vi "InitializePanelValues.vi"(11 "Experiment State in":T1={"error"={"status"=FALSE, "code"=0, "source"=""}, "Digitizer DAQmx Tasks"={"TaskArray"=[]}, "Digitizer Settings"={"Channel Settings"=[], "Card Settings"=[]}, "Synchronization Settings"={"Synchronizer 0"="", "source terminal"="", "Synchronizer 1"="PXI1Slot2"}, "Digitizer Data"=[], "Next Shot#"="", "System Message"="", "User Shot Notes"="", "Timing Settings"={"Timing Card Settings"=[], "Timing Channel Settings"=[]}, "Timing Tasks"={"TaskArray"=[]}, "Tree"="", "Time Card/Channels"=[], "DAQ Card/Channels"=[], "Program Version"="", "RIO Settings"={"Channel Settings"=[], "Card Settings"=[]}, "RIO References"={"Reference Array"=[]}, "RIO Data"={"RIO Deleaved Data"=[], "Raw Readout"=[]}} {"RIO Settings"."Card Settings"."Sample Rate" format="%#_3p"; "Timing Settings"."Timing Channel Settings"."FrontPanelTime" format="%.3p"; "Timing Settings"."Timing Channel Settings"."Pulse width (s)" format="%.3p"; "Timing Settings"."Timing Channel Settings"."Delay (s)" format="%.3p"; "Digitizer Settings"."Card Settings"."Global Edge Type" items=["Rising"=10280, "Falling"=10171]; "Digitizer Settings"."Card Settings"."Sample Rate" format="%#_3p"}) -> (0 "Initialized DAQ Array":T19(array[cluster]) {"Card Settings"."Start Time" format="%#_3p"; "Card Settings"."End Time" format="%#_3p"; "Card Settings"."Rate" format="%#_3p"}, 1 "Initialized Timing Array":T14[](array[typedef]) {"Timing Sequence"."Dt" format="%_3p"; "Timing Sequence"."Time" format="%_3p"}, 3 "Experiment State out":T1={"error"={"status"=FALSE, "code"=0, "source"=""}, "Digitizer DAQmx Tasks"={"TaskArray"=[]}, "Digitizer Settings"={"Channel Settings"=[], "Card Settings"=[]}, "Synchronization Settings"={"Synchronizer 0"="", "source terminal"="", "Synchronizer 1"="PXI1Slot2"}, "Digitizer Data"=[], "Next Shot#"="", "System Message"="", "User Shot Notes"="", "Timing Settings"={"Timing Card Settings"=[], "Timing Channel Settings"=[]}, "Timing Tasks"={"TaskArray"=[]}, "Tree"="", "Time Card/Channels"=[], "DAQ Card/Channels"=[], "Program Version"="", "RIO Settings"={"Channel Settings"=[], "Card Settings"=[]}, "RIO References"={"Reference Array"=[]}, "RIO Data"={"RIO Deleaved Data"=[], "Raw Readout"=[]}} {"RIO Settings"."Card Settings"."Sample Rate" format="%#_3p"; "Timing Settings"."Timing Channel Settings"."FrontPanelTime" format="%.3p"; "Timing Settings"."Timing Channel Settings"."Pulse width (s)" format="%.3p"; "Timing Settings"."Timing Channel Settings"."Delay (s)" format="%.3p"; "Digitizer Settings"."Card Settings"."Global Edge Type" items=["Rising"=10280, "Falling"=10171]; "Digitizer Settings"."Card Settings"."Sample Rate" format="%#_3p"}, 4 "Next Shot #":i32, 6 "System Message":string, 8 "Program Version":string)   [LabVIEW 2014]
doc: "Initialize values of various front panel boxes. Also initialized is the timing and DAQ card sequencers."
uses:
  Controls/ExperimentStateCluster.ctl
  Controls/DigitizerSettingsChannelSettings.ctl
  Controls/DigitizerSettingsCardSettingsArray.ctl
  Controls/DigitizerSettingsCardSettings.ctl
  Controls/TimingSettings.ctl
  Controls/TimingCardSettings.ctl
  Controls/TimingChannelSettings.ctl
  Controls/RIOSettingsExperimentStateCluster.ctl
  Controls/RIOSettingsChannelSettings.ctl
  Controls/RIOSettingsCardSettingsArray.ctl
  Controls/RIOSettingsCardSettings.ctl
  <vilib>/userdefined/High Color/nirio_resource_hc.ctl
  Controls/RIOData.ctl
  Controls/DAQ Card Channel Array.ctl
  Controls/DAQ Channel Settings.ctl
  Controls/DAQ Card Settings.ctl
  Controls/TimingControl.ctl
  Controls/TimingControlChannel.ctl
panel:
  # "Sampling Rate [1/s]"
  # "Start Time [s]"
  # "End Time [s]"
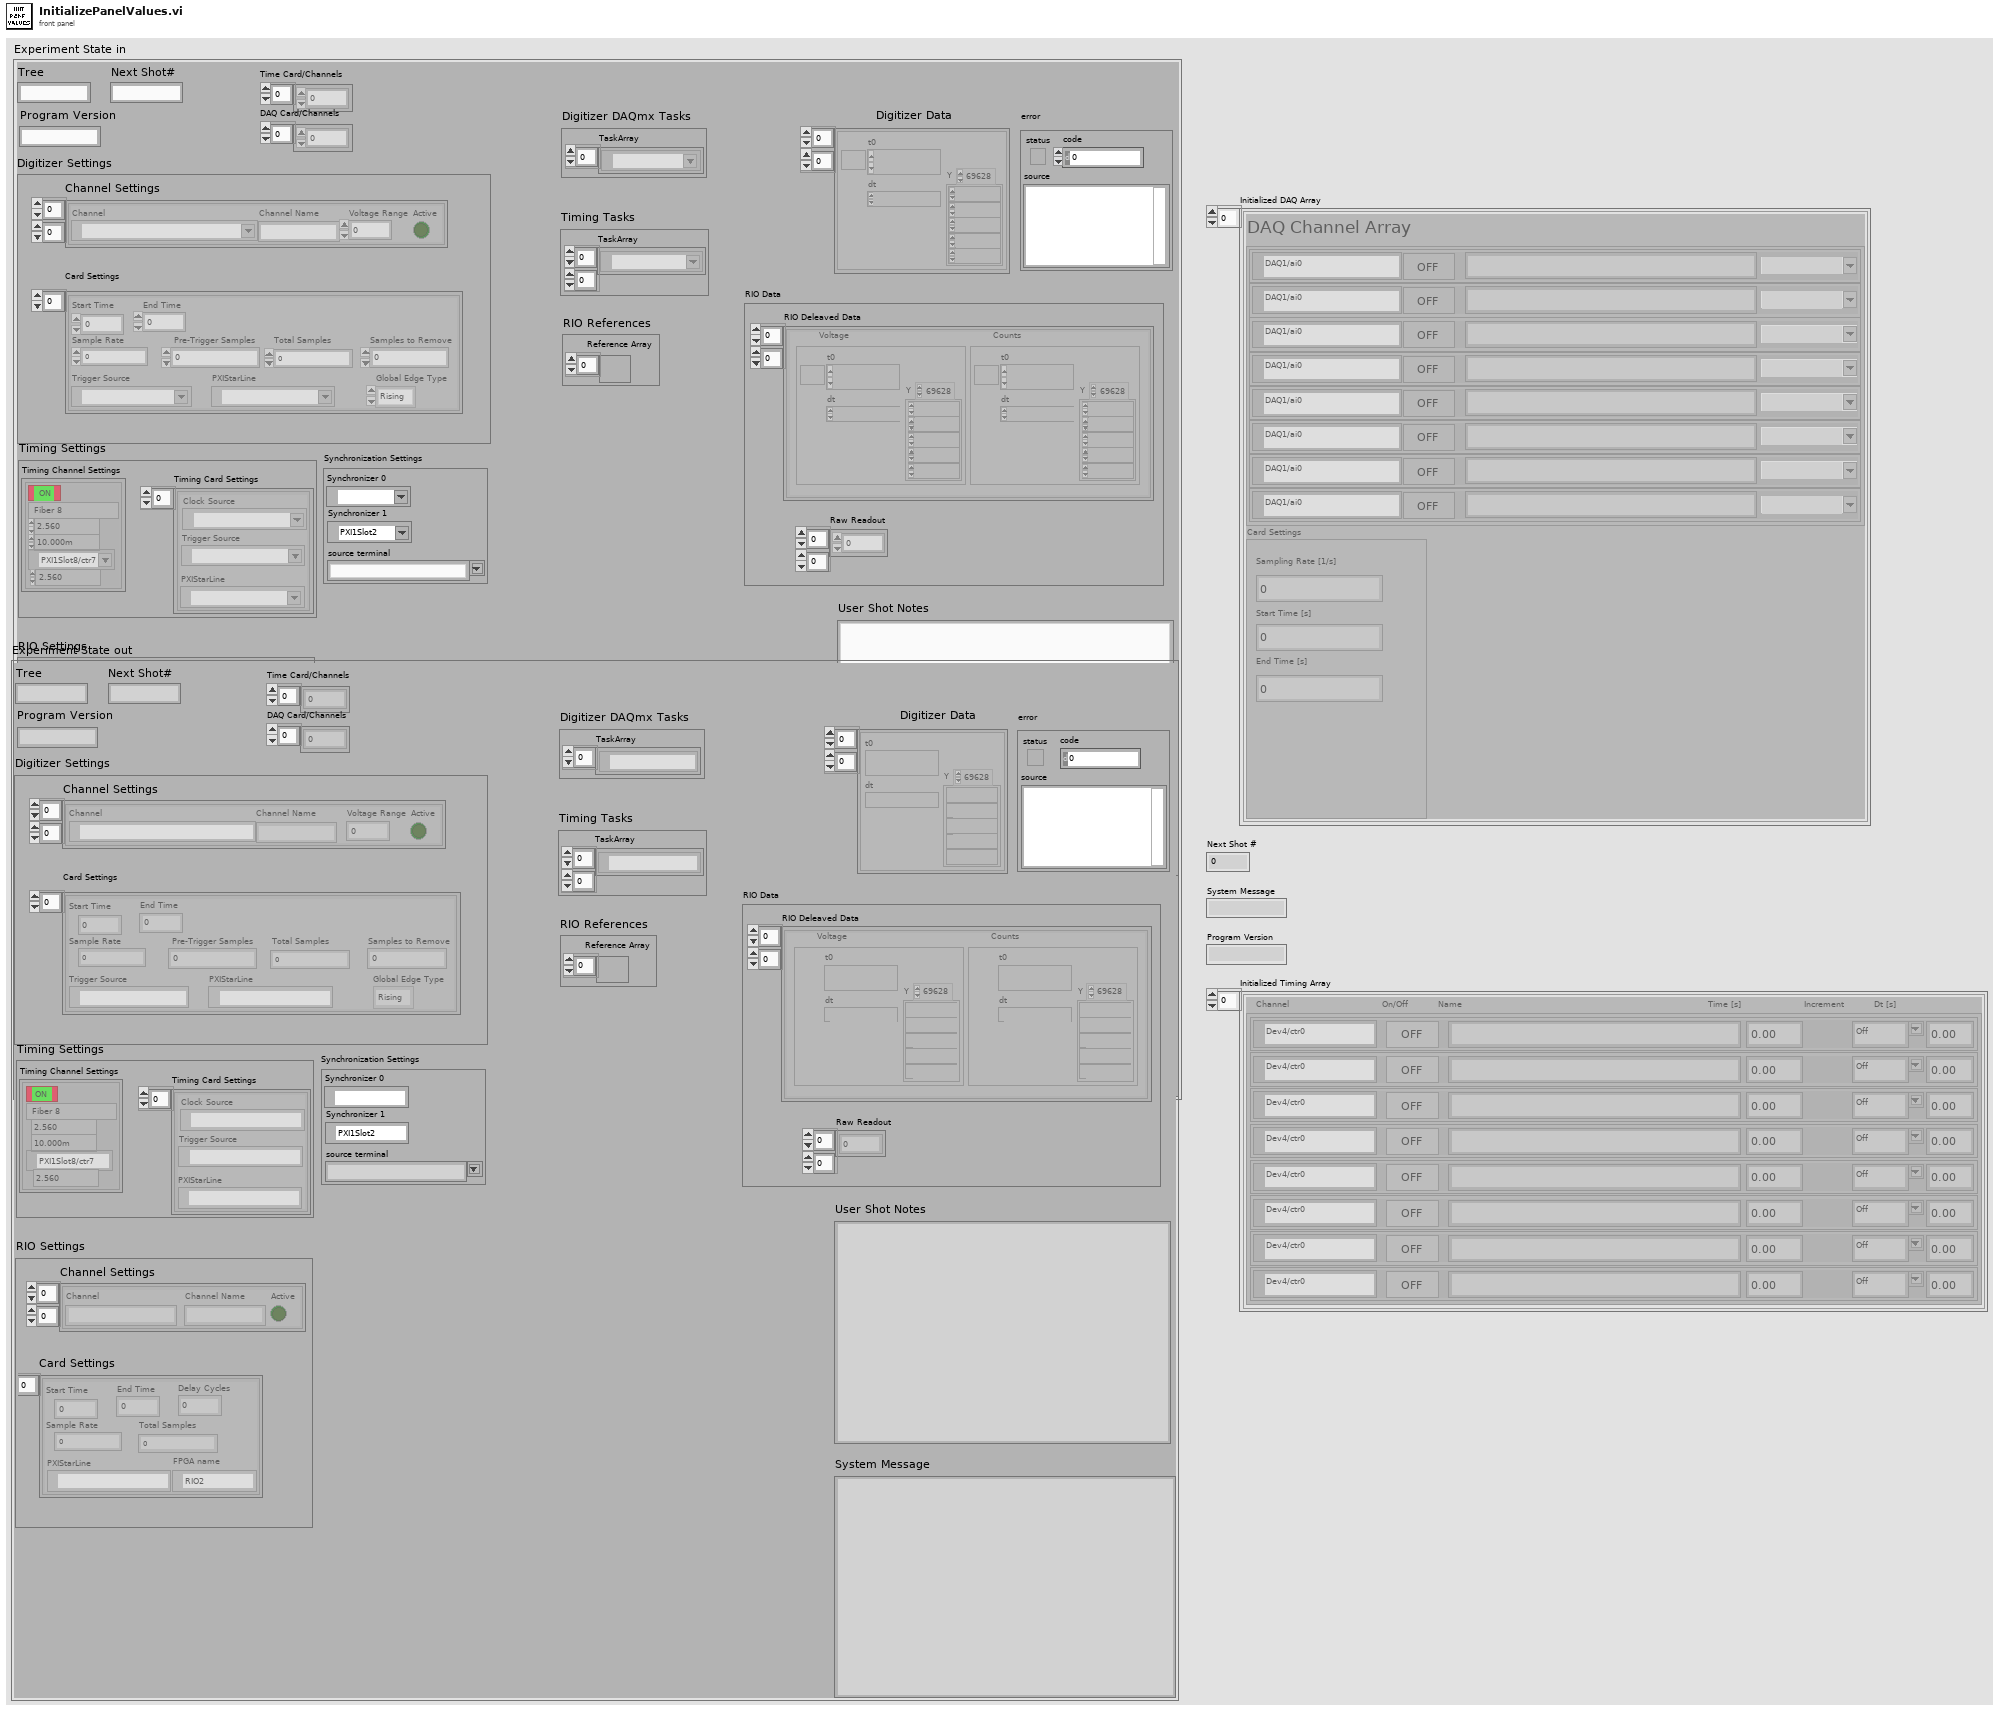
[diagram p1: front panel]
types:
  T1 = typedef "ExperimentStateCluster.ctl" = cluster{"error":errorcluster, "Digitizer DAQmx Tasks":cluster{"TaskArray":refnum<k21>[]}, "Digitizer Settings":cluster{"Channel Settings":T2[][], "Card Settings":T3}, "Synchronization Settings":cluster{"Synchronizer 0":refnum<k15>, "source terminal":string, "Synchronizer 1":refnum<k15>}, "Digitizer Data":waveform(dbl)[][], "Next Shot#":string, "System Message":string, "User Shot Notes":string, "Timing Settings":T5, "Timing Tasks":cluster{"TaskArray":refnum<k21>[][]}, "Tree":string, "Time Card/Channels":i32[], "DAQ Card/Channels":i32[], "Program Version":string, "RIO Settings":T8, "RIO References":cluster{"Reference Array":refnum<k20>[]}, "RIO Data":T13}
  T2 = typedef "DigitizerSettingsChannelSettings.ctl" = cluster{"Channel":tag, "Channel Name":string, "Voltage Range":dbl, "Active":bool}
  T3 = typedef "DigitizerSettingsCardSettingsArray.ctl" = T4[]
  T4 = typedef "DigitizerSettingsCardSettings.ctl" = cluster{"Start Time":dbl, "End Time":dbl, "Sample Rate":dbl, " Pre-Trigger Samples":u32, "Total Samples":i32, "Samples to Remove":u32, "Trigger Source":tag, "Global Edge Type":i32, "PXIStarLine":tag}
  T5 = typedef "TimingSettings.ctl" = cluster{"Timing Card Settings":T6[], "Timing Channel Settings":T7[][]}
  T6 = typedef "TimingCardSettings.ctl" = cluster{"Trigger Source":tag, "Clock Source":tag, "PXIStarLine":tag}
  T7 = typedef "TimingChannelSettings.ctl" = cluster{"Delay (s)":dbl, "Pulse width (s)":dbl, "Active":bool, "Channel Name":string, "counter":tag, "FrontPanelTime":dbl}
  T8 = typedef "RIOSettingsExperimentStateCluster.ctl" = cluster{"Channel Settings":T9[][], "Card Settings":T10}
  T9 = typedef "RIOSettingsChannelSettings.ctl" = cluster{"Channel Name":string, "Active":bool, "Channel":string}
  T10 = typedef "RIOSettingsCardSettingsArray.ctl" = T11[]
  T11 = typedef "RIOSettingsCardSettings.ctl" = cluster{"Start Time":dbl, "End Time":dbl, "Sample Rate":dbl, "Total Samples":u64, "PXIStarLine":tag, "Delay Cycles":u64, "FPGA name":T12}
  T12 = typedef "nirio_resource_hc.ctl" = tag
  T13 = typedef "RIOData.ctl" = cluster{"RIO Deleaved Data":cluster{"Voltage":waveform(dbl), "Counts":waveform(i16)}[][], "Raw Readout":u64[][]}
  T14 = typedef "TimingControl.ctl" = cluster{"Timing Sequence":T15[]}
  T15 = typedef "TimingControlChannel.ctl" = cluster{"Active":bool, "counter":tag, "Channel Name":string, "Time":dbl, "Increment":string, "Dt":dbl}
  T16 = typedef "DAQ Card Channel Array.ctl" = T17[]
  T17 = typedef "DAQ Channel Settings.ctl" = cluster{"Active":bool, "Channel Name":string, "Channel":tag, "Voltage Range":string}
  T18 = typedef "DAQ Card Settings.ctl" = cluster{"Rate":dbl, "End Time":dbl, "Start Time":dbl}
  T19 = cluster{"DAQ Channel Array":T16, "Card Settings":T18}[]
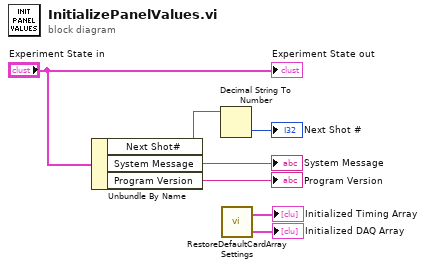
[diagram p0: block diagram]
diagram:
  n1 = Unbundle By Name("Experiment State in") -> ("Next Shot#"=w3:string, "System Message"=→"System Message":string, "Program Version"=→"Program Version":string)
  n2 = Decimal String To Number(string=w3) -> (number=→"Next Shot #":i32)  [unwired: 2 in, 1 out]
  n3 = call "RestoreDefaultCardArraySettings.vi"() -> ("Initialized DAQ Array"=→"Initialized DAQ Array":T19, "Initialized Timing Array"=→"Initialized Timing Array":T14[])  [unwired: 2 in]
  "Experiment State out" <- "Experiment State in"
